vi "Labview HW2_sol.vi"() -> ()   [LabVIEW 2019]
panel:
  out "Waveform Graph":dynamicdata(graph)
  in  "Square Offset":dbl
  in  "square Frequency":dbl
  in  "square Amplitude":dbl
  in  "Sine Offset":dbl
  in  "Sine Phase":dbl
  in  "Sine Frequency":dbl
  in  "Sine Amplitude":dbl
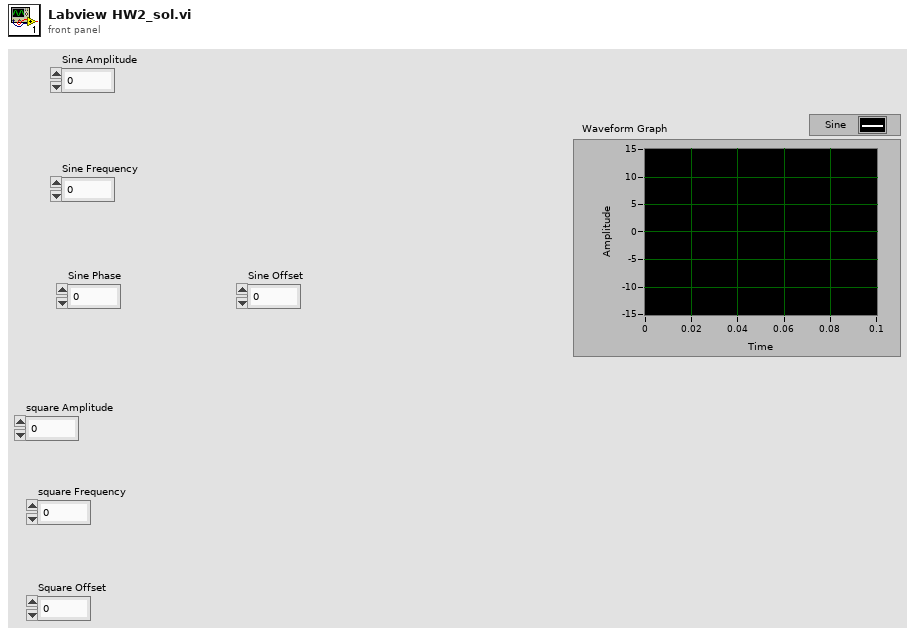
[diagram p1: front panel]
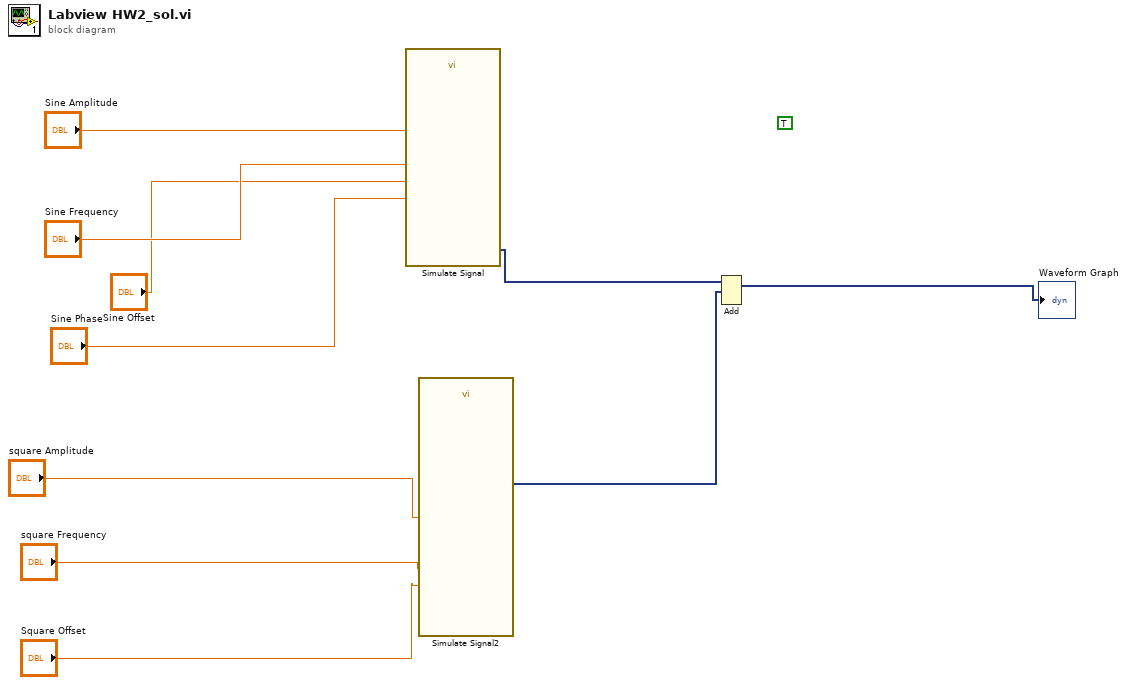
[diagram p0: block diagram]
diagram:
  (unwired) TRUE
  n1 = call "Simulate Signal"("Offset"="Sine Offset", "Frequency"="Sine Frequency", "Amplitude"="Sine Amplitude", "Phase"="Sine Phase") -> ("Sine"=w3:dynamicdata)  [unwired: 10 in, 1 out]
  n2 = call "Simulate Signal2"("Offset"="Square Offset", "Frequency"="square Frequency", "Amplitude"="square Amplitude") -> ("Square"=w2:dynamicdata)  [unwired: 11 in, 1 out]
  n3 = Add(1:w2, 2:w3) -> (0:→"Waveform Graph":dynamicdata)  [unwired: 1 in, 1 out]
